vi "DjtgGetPortProperties.vi"(8 "Error In":errorcluster, 10 "Port Number":i32, 11 "Device Number":u32) -> (0 "Error Out":errorcluster, 2 "Port Properties":T1, 3 "Device Number":u32)   [LabVIEW 2011, in "LVH-Adept.lvlib" / "DJTG.lvlib"]
doc: "This function returns the port properties bits for the specified DJTG port. The port properties bits\nindicate the specific features of the DJTG specification implemented by the specified port."
uses:
  <vilib>/LabVIEW Hacker/Adept/Private/DJTG/DJTG.lvlib
  <vilib>/LabVIEW Hacker/Adept/Private/DJTG/Private/Type Defs/Port Properties.ctl
  <vilib>/LabVIEW Hacker/Adept/Private/DJTG/Private/Type Defs/Error.ctl
  <vilib>/LabVIEW Hacker/Adept/Private/Resources/djtg.dll
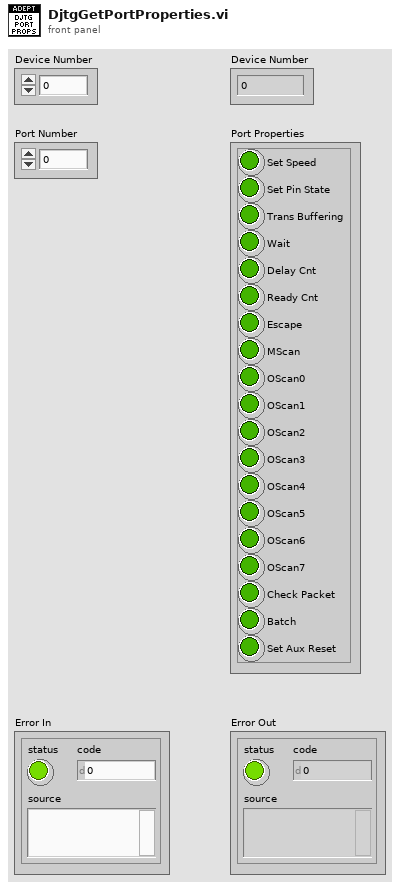
[diagram p1: front panel]
types:
  T1 = typedef "LVH-Adept.lvlib/DJTG.lvlib/Port Properties.ctl" = cluster{"Set Speed":bool, "Set Pin State":bool, "Trans Buffering":bool, "Wait":bool, "Delay Cnt":bool, "Ready Cnt":bool, "Escape":bool, "MScan":bool, "OScan0":bool, "OScan1":bool, "OScan2":bool, "OScan3":bool, "OScan4":bool, "OScan5":bool, "OScan6":bool, "OScan7":bool, "Check Packet":bool, "Batch":bool, "Set Aux Reset":bool}
  T2 = typedef "LVH-Adept.lvlib/DJTG.lvlib/Error.ctl" = enum16{"Unknown", "Enable", "PutTmsTdiBits", "GetTdoBits", "Disable", "Close", "Set Aux Reset", "Port Properties", "Get Speed", "Set Speed", "Get Port Count", "Get Batch Properties", "Enable Port", "Set Tmd Tdi Tck", "Get Tms Tdi Tdo Tck", "Put Tdi Bits", "Put Tms Bits", "Clock Tck", "Wait", "Batch", "Flash FPGA"}
  T3 = cluster{"Boolean array[0]":bool, "Boolean array[1]":bool, "Boolean array[2]":bool, "Boolean array[3]":bool, "Boolean array[4]":bool, "Boolean array[5]":bool, "Boolean array[6]":bool, "Boolean array[7]":bool, "Boolean array[8]":bool}
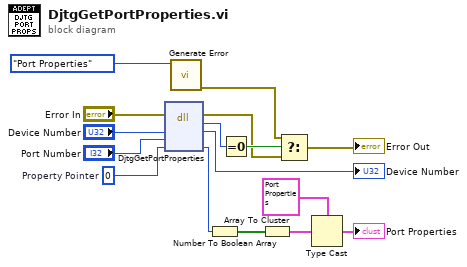
[diagram p0: block diagram]
diagram:
  w6 = u32 0  # Property Pointer
  n1 = dll-call lib="C:/Program Files (x86)/National Instruments/LabVIEW 2011/vi.lib/LabVIEW Hacker/Adept/Private/Resources/djtg.dll" fn="DjtgGetPortProperties"(error in="Error In", "HIF"="Device Number", "prtReq"="Port Number", "pdprp"=w6) -> (error out=w12:errorcluster, "Success"=w14:u32, "HIF"=→"Device Number":u32, "pdprp"=w1:u32)  [unwired: 3 in, 1 out]
  n2 = call <vilib>:"Generate Error.vi"("DJTG Error"=Error."Port Properties") -> ("Error Out"=w13:errorcluster)  [unwired: 10 in]
  n3 = Number To Boolean Array(number=w1) -> (Boolean array=w4:bool[])
  n4 = Equal To 0?(x=w14) -> (x = 0?=w15:bool)
  n5 = Array To Cluster(array=w4) -> (cluster=w3:T3)
  n6 = Select(t=w13, s=w15, f=w12) -> (s? t:f=→"Error Out":errorcluster)
  n7 = Type Cast(type=T1 {"Set Speed"=FALSE, "Set Pin State"=FALSE, "Trans Buffering"=FALSE, "Wait"=FALSE, "Delay Cnt"=FALSE, "Ready Cnt"=FALSE, "Escape"=FALSE, "MScan"=FALSE, "OScan0"=FALSE, "OScan1"=FALSE, "OScan2"=FALSE, "OScan3"=FALSE, "OScan4"=FALSE, "OScan5"=FALSE, "OScan6"=FALSE, "OScan7"=FALSE, "Check Packet"=FALSE, "Batch"=FALSE, "Set Aux Reset"=FALSE} ("Port Properties"), x=w3) -> (*(type *) &x=→"Port Properties":T1)
